vi "main 2.18.22.vi"() -> ()   [LabVIEW 2021]
uses:
  <vilib>/ptbypt/NI_PtbyPt.lvlib
  <vilib>/express/express arith-compare/Formula/XNode/ExpressFormulaBlockNode.xnode
panel:
  out "Thermistor Filtered":dbl[](graph)
  out "Thermistor Unfiltered":dbl[](graph)
  in  "Thermistor":T1
  out "Waveform Chart 3":T2(graph)
  in  "error in (no error)":errorcluster
  out "error out":errorcluster
  out "Waveform Chart 2":waveform(dbl)(graph)
  out "a0 Scalar":dbl
  out "Waveform Chart":dynamicdata(graph)
  in  "stop":bool
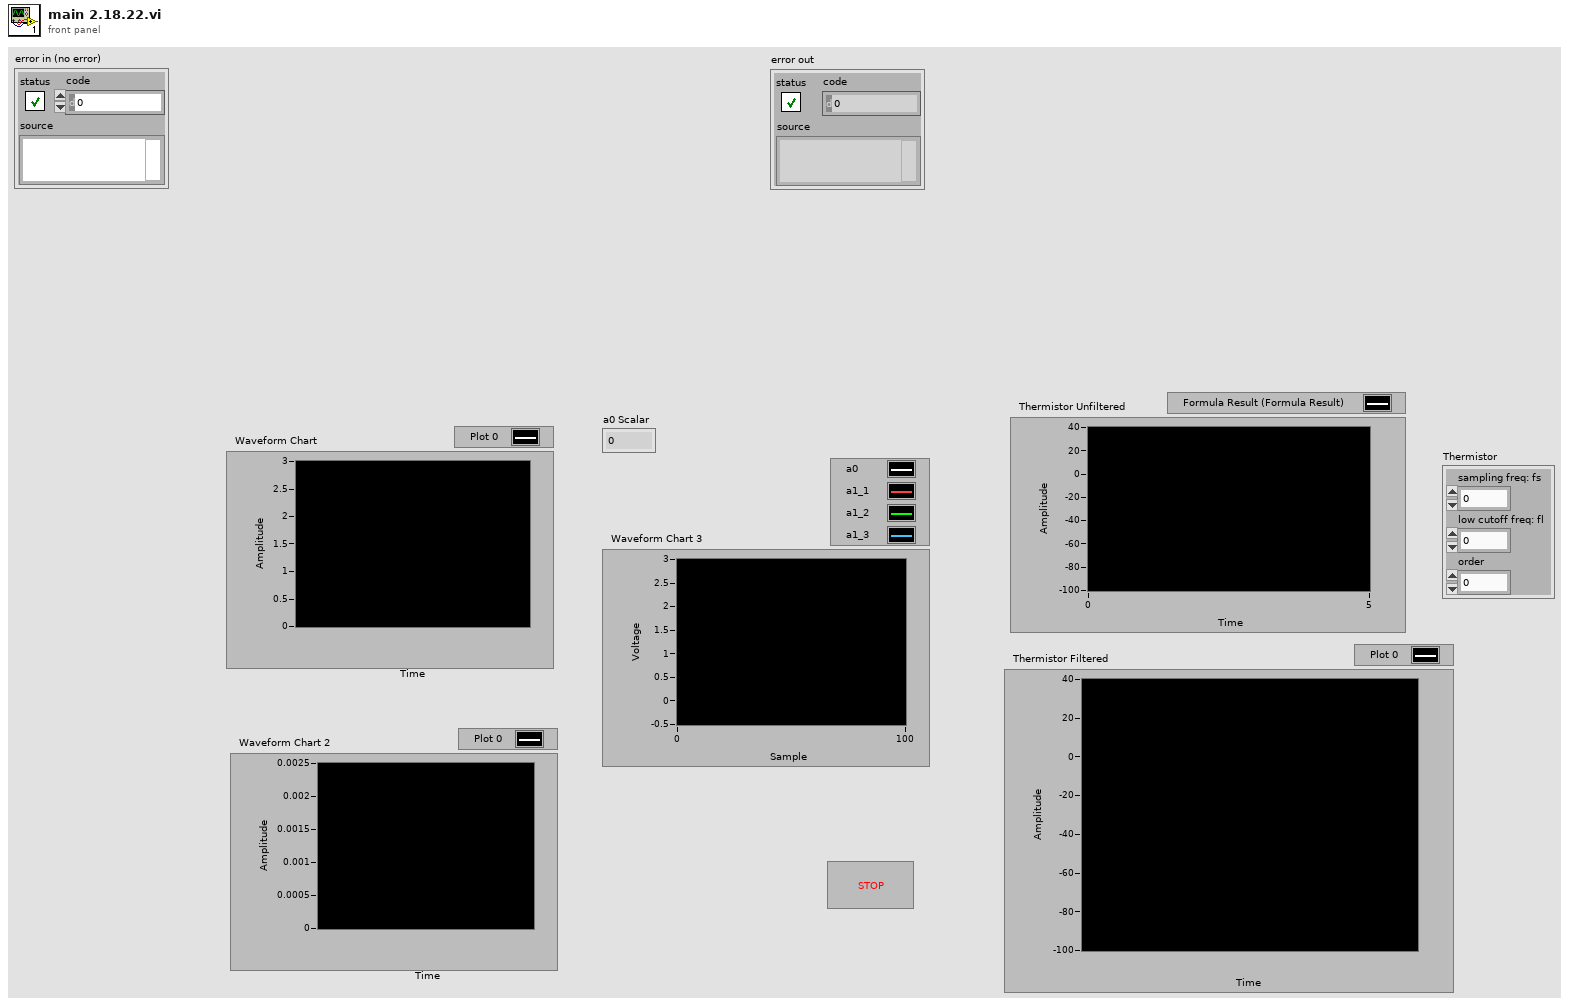
[diagram p1: front panel]
types:
  T1 = cluster{"sampling freq: fs":dbl, "low cutoff freq: fl":dbl, "order":i32}
  T2 = cluster{"Data_Array[0]":dbl, "Data_Array[1]":dbl, "Data_Array[2]":dbl, "Data_Array[3]":dbl, "Data_Array[4]":dbl, "Data_Array[5]":dbl, "Data_Array[6]":dbl, "Data_Array[7]":dbl, "Data_Array[8]":dbl}
  T3 = cluster{"Data_Array":dbl[], "Multiplex_Tbl":u32[]}
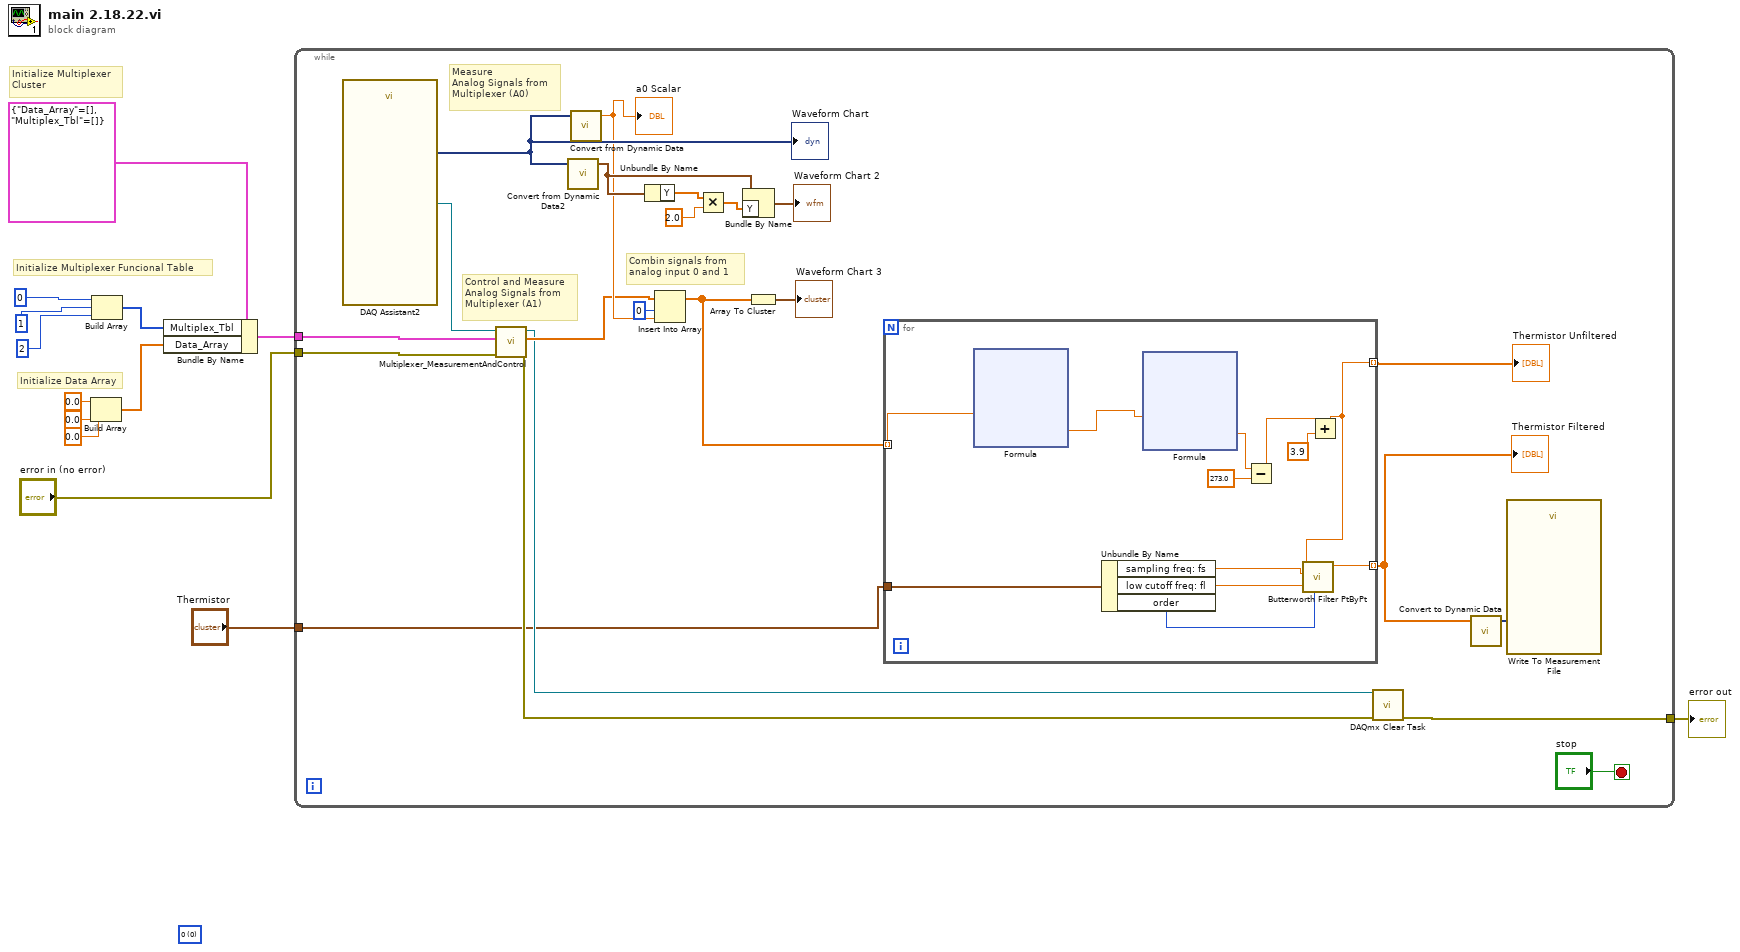
[diagram p0: block diagram]
diagram:
  (unwired) u8 0 items=["0", "1", "Z", "L", "H", "X", "T", "V"] ("digital values ring")
  # "Initialize Multiplexer \nCluster"
  # "Initialize Data Array"
  # "Initialize Multiplexer Funcional Table"
  n1 = Build Array(0.0 ("element"), 0.0 ("element"), 0.0 ("element")) -> (w9:dbl[])
  n2 = Build Array(u32 0 ("Waveform"), 1 ("Waveform"), u32 2 ("Waveform")) -> (w3:u32[])
  n3 = Bundle By Name(cluster=T3 {"Data_Array"=[], "Multiplex_Tbl"=[]}, "Multiplex_Tbl"=w3, "Data_Array"=w9) -> (w8:T3)
  n4 = while {
    tunnel: w8 -> [w28]
    tunnel: "error in (no error)" -> [w27]
    tunnel: [w19] -> w2
    tunnel: "Thermistor" -> [w18]
    stop <- "stop" stop-if-true
    # "Combin signals from \nanalog input 0 and 1"
    # "Measure\nAnalog Signals from\nMultiplexer (A0)"
    # "Control and Measure\nAnalog Signals from\nMultiplexer (A1)"
    n5 = call "DAQ Assistant2"() -> ("task out"=w26:refnum<k21>, "data"=w29:dynamicdata)  [unwired: 16 in, 2 out]
    "Waveform Chart" <- w29
    n6 = call "Multiplexer_MeasurementAndControl.vi"("error in (no error)"=w27, "Multiplexer_Cluser"=w28, "Task in"=w26) -> ("error out"=w20:errorcluster, "Data_Array"=w23:dbl[], "Task out"=w21:refnum<k21>)  [unwired: 6 in]
    n7 = call "Convert from Dynamic Data2"("Dynamic Data Type"=w29) -> ("Waveform"=w32:waveform(dbl))  [unwired: 3 in]
    n8 = call "Convert from Dynamic Data"("Dynamic Data Type"=w29) -> ("Scalar"=w25:dbl)  [unwired: 3 in]
    "a0 Scalar" <- w25
    n9 = Unbundle By Name(w32) -> ("Y"=w34:dbl[])
    n10 = Insert Into Array(array=w23, index=0, new element=w25) -> (w17:dbl[])
    n11 = Multiply(x=w34, y=2.0) -> (x*y=w31:dbl[])
    n12 = Bundle By Name(cluster=w32, "Y"=w31) -> (→"Waveform Chart 2":waveform(dbl))
    n13 = Array To Cluster(array=w17) -> (cluster=→"Waveform Chart 3":T2)
    n14 = for {
      tunnel: w17 -> [w39] mode=indexing
      tunnel: w18 -> [w38]
      tunnel: [w37] -> w15 mode=indexing
      tunnel: [w36] -> w14 mode=indexing
      n15 = xnode "Formula"("v"=w39) -> ("Result"=w46:dbl)  [unwired: 1 in, 1 out]
      n16 = Unbundle By Name(w38) -> ("sampling freq: fs"=w45:dbl, "low cutoff freq: fl"=w44:dbl, "order"=w43:i32)
      n17 = xnode "Formula"("R"=w46) -> ("Result"=w41:dbl)  [unwired: 1 in, 1 out]
      n18 = Subtract(x=w41, y=273.0) -> (x-y=w40:dbl)
      n19 = Add(x=w40, y=3.9) -> (x+y=w37:dbl)
      n20 = call <vilib>:"Butterworth Filter PtByPt.vi"("order"=w43, "low cutoff freq: fl"=w44, "sampling freq: fs"=w45, "x"=w37) -> ("Filtered x"=w36:dbl)  [unwired: 5 in, 1 out]
    }
    "Thermistor Unfiltered" <- w15
    "Thermistor Filtered" <- w14
    n21 = call <vilib>:"DAQmx Clear Task.vi"("task in"=w21, "error in"=w20) -> ("error out"=w19:errorcluster)  [unwired: 13 in]
    n22 = call "Convert to Dynamic Data"("Array"=w14) -> ("Dynamic Data Type"=w16:dynamicdata)  [unwired: 3 in]
    n23 = call "Write To Measurement File"("Signals"=w16) -> ()  [unwired: 16 in, 3 out]
  }
  "error out" <- w2
